vi "ObtainMsgQueue.vi"(8 "ErrorArray In":errorcluster[](array[cluster])) -> (0 "ErrorArray Out":errorcluster[](array[cluster]), 3 "QueRef":T1)   [LabVIEW 2014, in "TestFramework.lvlib"]
uses:
  TestFramework.lvlib
  TypeDef/QueRef.ctl
  TypeDef/MsgQueue.ctl
  <userlib>/NIST/NISTErrorLib/NISTErrorLib.lvlib
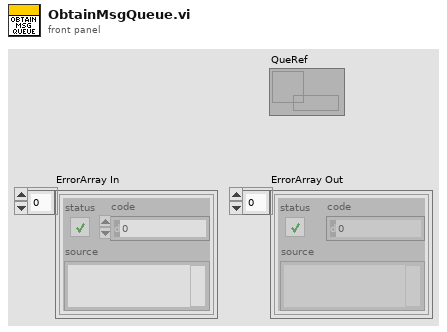
[diagram p1: front panel]
types:
  T1 = typedef "TestFramework.lvlib/QueRef.ctl" = refnum<queue>
  T2 = typedef "TestFramework.lvlib/MsgQueue.ctl" = cluster{"Msg":string, "Data":variant}
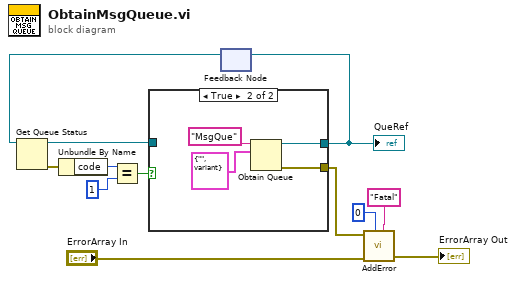
[diagram p0: block diagram]
diagram:
  n1 = feedback #1() -> (w7:refnum<queue>)  [unwired: 1 in]
  n2 = Get Queue Status(queue=w7) -> (queue out=w6:refnum<queue>, error out=w5:errorcluster)  [unwired: 2 in, 6 out]
  n3 = Unbundle By Name(w5) -> ("code"=w3:i32)
  n4 = Equal?(x=w3, y=1) -> (x = y?=w4:bool)
  n5 = case shown="True" w4 {
    tunnel: [w13 w15] -> w8
    tunnel: [_ w14] -> w1
    tunnel: w6 -> [w13 _]
    frame False {
    }
    frame True {
      n6 = Obtain Queue(name (unnamed)="MsgQue", element data type=T2 {"Msg"="", "Data"=variant} ("MsgQueue")) -> (queue out=w15:refnum<queue>, error out=w14:errorcluster)  [unwired: 3 in, 1 out]
    }
  }
  "QueRef" <- w8
  n7 = feedback-in #1(w8) -> ()
  n8 = call <userlib>:"AddError.vi"("Severity"="Fatal", "Priority"=u8 0, "ErrorArray"="ErrorArray In", "error in (no error)"=w1) -> ("ErrorArray"=→"ErrorArray Out":errorcluster[])  [unwired: 6 in, 1 out]
